vi "Protocol Factory.vi"(8 "error in (no error)":errorcluster, 10 "Protocol":enum16{"RS-xxx", "TCP", "UDP", "VISA"}(ring)) -> (0 "error out":errorcluster, 3 "Protocol Out":refnum<class "Protocol Parent.lvclass">)   [LabVIEW 2019]
uses:
  Protocol Parent/Protocol Parent.lvclass
  RS-xxx/RS-xxx.lvclass
  C:/Dev/niveristand-instrument-addon-classes/Source/Protocols/Protocol Parent/Protocol Parent.lvclass
  TCP/TCP.lvclass
  UDP/UDP.lvclass
  VISA/VISA.lvclass
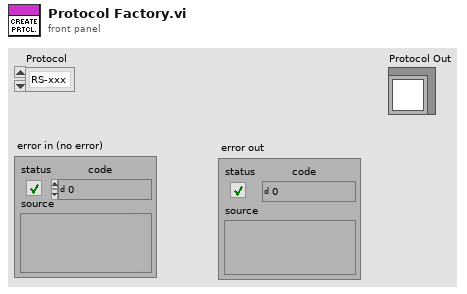
[diagram p1: front panel]
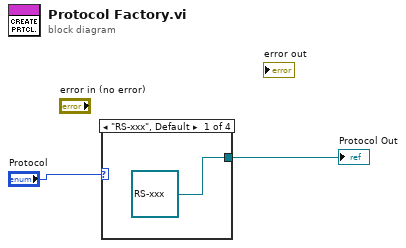
[diagram p0: block diagram]
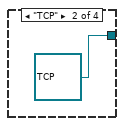
[diagram p2: hidden frame]
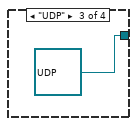
[diagram p3: hidden frame]
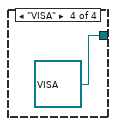
[diagram p4: hidden frame]
diagram:
  n1 = case shown="\"RS-xxx\", Default" "Protocol" {
    tunnel: [refnum<class "RS-xxx.lvclass"> refnum ("Protocols.lvlib:RS-xxx.lvclass") refnum<class "TCP.lvclass"> refnum ("Protocols.lvlib:TCP.lvclass") refnum<class "UDP.lvclass"> refnum ("Protocols.lvlib:UDP.lvclass") refnum<class "VISA.lvclass"> refnum ("Protocols.lvlib:VISA.lvclass")] -> w1
    frame "RS-xxx", Default {
    }
    frame "TCP" {
    }
    frame "UDP" {
    }
    frame "VISA" {
    }
  }
  "Protocol Out" <- w1
